vi "StopSubsystem.vi"(8 "error in (no error)":errorcluster, 11 "DriveAuto in":refnum<class "DriveAuto.lvclass">) -> (0 "error out":errorcluster, 3 "DriveAuto out":refnum<class "DriveAuto.lvclass">)   [LabVIEW 2017, in "DriveAuto.lvclass"]
uses:
  DriveAuto.lvclass
  AutoSubsystem/AutoSubroutine.lvclass
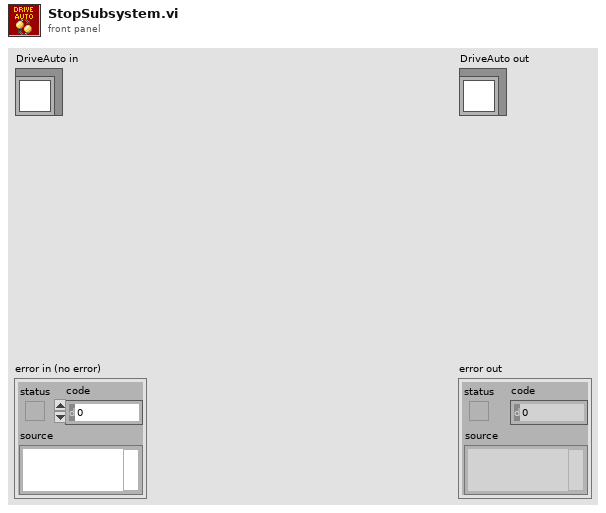
[diagram p1: front panel]
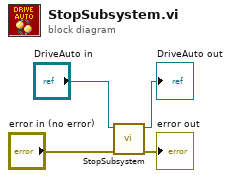
[diagram p0: block diagram]
diagram:
  n1 = call-parent "StopSubsystem.vi"("error in (no error)"="error in (no error)", "AutoSubroutine in"="DriveAuto in") -> ("error out"=→"error out":errorcluster, "AutoSubroutine out"=→"DriveAuto out":refnum<class "DriveAuto.lvclass">)  [unwired: 8 in]
